vi "Insert In Reference Cache.vi"(8 "error in (no error)":errorcluster, 9 "Variant":variant, 10 "VIQualifiedName":string, 11 "App Control API in":refnum<class "AppControlAPI.lvclass">) -> (0 "error out":errorcluster, 3 "App Control API out":refnum<class "AppControlAPI.lvclass">)   [LabVIEW 2018, in "AppControlAPI.lvclass"]
uses:
  AppControlAPI.lvclass
  AppControlAPI.lvclass/AppControlAPI.ctl
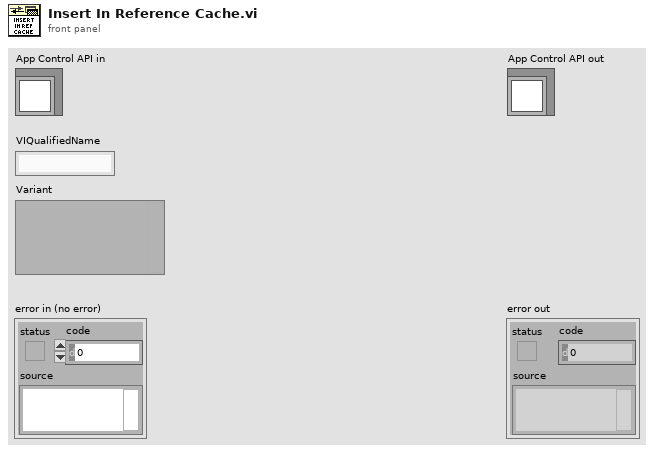
[diagram p1: front panel]
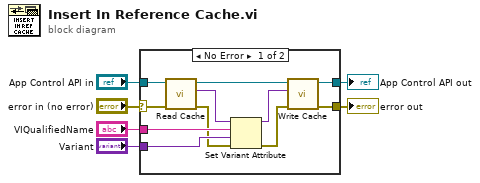
[diagram p0: block diagram]
diagram:
  n1 = case shown="No Error" "error in (no error)" {
    selector: "error in (no error)" -> [w14 w19]
    tunnel: [w13 w19] -> w5
    tunnel: [w12 w18] -> w3
    tunnel: "App Control API in" -> [w15 w18]
    tunnel: "VIQualifiedName" -> [w17 _]
    tunnel: "Variant" -> [w16 _]
    frame No Error {
      n2 = call "Read Cache.vi"("error in (no error)"=w14, "App Control API in"=w15) -> ("error out"=w11:errorcluster, "Cache"=w9:variant, "App Control API out"=w10:refnum<class "AppControlAPI.lvclass">)  [unwired: 7 in]
      n3 = Set Variant Attribute(Variant=w9, name=w17, value=w16, error in=w11) -> (Variant out=w8:variant, error out=w7:errorcluster)  [unwired: 1 out]
      n4 = call "Write Cache.vi"("error in (no error)"=w7, "Cache"=w8, "App Control API in"=w10) -> ("error out"=w13:errorcluster, "App Control API out"=w12:refnum<class "AppControlAPI.lvclass">)  [unwired: 7 in]
    }
    frame Error {
    }
  }
  "error out" <- w5
  "App Control API out" <- w3
